vi "NormalizeJoystick.vi"(1 "joystick":cluster{"X":dbl, "Y":dbl}) -> (0 "normalized joystick":cluster{"x":dbl, "y":dbl})   [LabVIEW 2014]
panel:
  out "Direction":dbl(knob) scale=3.1416..-3.1416
  out "Magnitude":dbl(slide) scale=-1.0..1.0
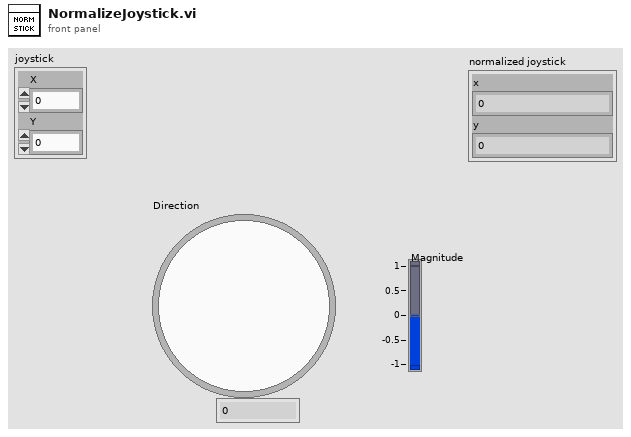
[diagram p1: front panel]
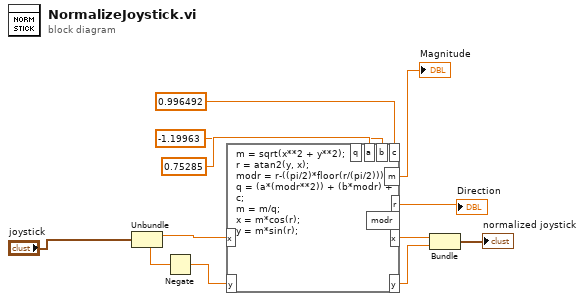
[diagram p0: block diagram]
diagram:
  n1 = Unbundle("joystick") -> ("X"=w7:dbl, "Y"=w8:dbl)
  n2 = Negate(x=w8) -> (-x=w12:dbl)
  n3 = formula code="m = sqrt(x**2 + y**2);\nr = atan2(y, x);\nmodr = r-((pi/2)*floor(r/(pi/2)));\nq = (a*(modr**2)) + (b*modr) + c;\nm = m/q;\nx = m*cos(r);\ny = m*sin(r);"("x"=w7, "y"=w12, "a"=0.75285, "b"=-1.19963, "c"=0.996492 ("value")) -> ("y"=w5:dbl, "x"=w6:dbl, "m"=→"Magnitude":dbl, "r"=→"Direction":dbl)  [unwired: 2 out]
  n4 = Bundle("x"=w6, "y"=w5) -> (→"normalized joystick":cluster{"x":dbl, "y":dbl})  [unwired: 1 in]
